vi "Check pre-empt -- Boolean.vi"(8 "error in (no error)":errorcluster, 11 "_Popup in":refnum<class "Popup.lvclass">) -> (0 "error out":errorcluster, 1 "Value?":bool, 2 "Pre-empted?":bool, 4 "Type Match?":bool)   [LabVIEW 2021, in "Pop-Up.lvlib" / "Popup.lvclass"]
doc: "check on the status of the pre-empt notifier\n\n<b>Code Developed By:</b> +\nDaniel Coons +\nhttps://github.com/danielcoons/tsc-pop-up"
uses:
  Popup.lvclass
  Popup.lvclass/Popup.ctl
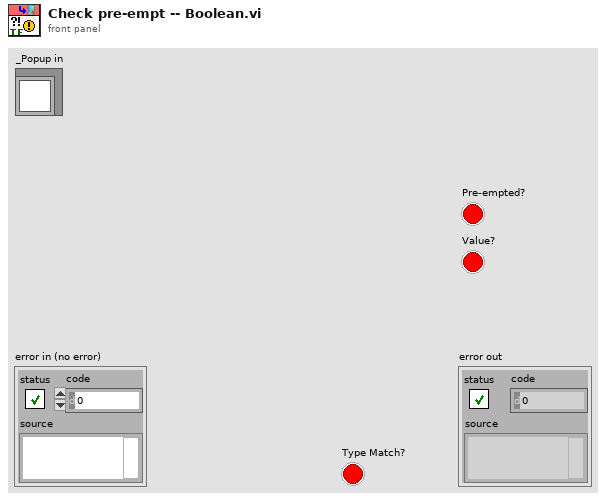
[diagram p1: front panel]
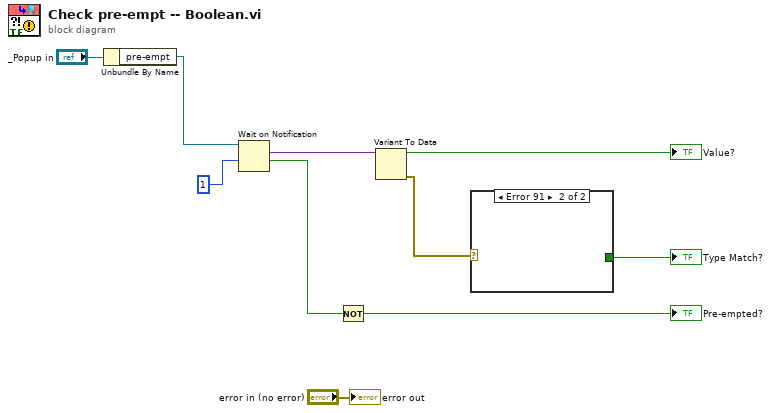
[diagram p0: block diagram]
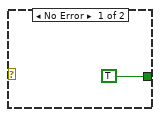
[diagram p2: hidden frame]
diagram:
  n1 = Unbundle By Name("_Popup in") -> ("pre-empt"=w8:refnum<notifier>)
  n2 = Wait on Notification(notifier=w8, timeout in ms (-1)=1) -> (notification=w4:variant, timed out?=w6:bool)  [unwired: 2 in, 2 out]
  n3 = Not(x=w6) -> (.not. x?=→"Pre-empted?":bool)
  n4 = Variant To Data(Variant=w4) -> (data=→"Value?":bool, error out=w1:errorcluster)  [unwired: 2 in]
  n5 = case shown="Error 91" w1 {
    tunnel: [TRUE _] -> w2
    frame No Error {
    }
    frame Error {
    }
  }
  "Type Match?" <- w2
  "error out" <- "error in (no error)"
